vi "WILT Search Agilent Label.vi"(8 "Error In":errorcluster, 9 "Array in":string[](array[string]), 10 "Search For":string, 11 "Agilent Channel Definition":T1) -> (0 "Error Out":errorcluster, 3 "Array out":string[](array[string]))   [LabVIEW 2016]
uses:
  Type Definitions/WILT Agilent Channel Definition.ctl
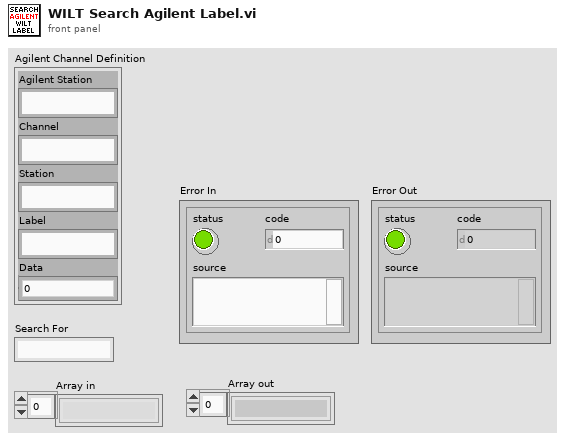
[diagram p1: front panel]
types:
  T1 = typedef "WILT Agilent Channel Definition.ctl" = cluster{"Channel":string, "Station":string, "Label":string, "Agilent Station":string, "Data":dbl}
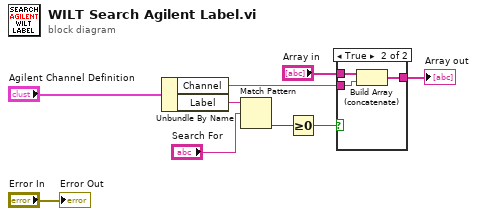
[diagram p0: block diagram]
diagram:
  n1 = Unbundle By Name("Agilent Channel Definition") -> ("Channel"=w7:string, "Label"=w8:string)
  n2 = Match Pattern(string=w8, regular expression="Search For") -> (offset past match=w3:i32)  [unwired: 1 in, 3 out]
  n3 = Greater Or Equal To 0?(x=w3) -> (x >= 0?=w2:bool)
  n4 = case shown="True" w2 {
    tunnel: w7 -> [_ w13]
    tunnel: [w10 w12] -> w5
    tunnel: "Array in" -> [w10 w11]
    frame False {
    }
    frame True {
      n5 = Build Array (concatenate)(w11, w13) -> (w12:string[])
    }
  }
  "Array out" <- w5
  "Error Out" <- "Error In"
